vi "Determine Warning Bad One.vi"(6 "High":dbl, 7 "wind":dbl, 8 "error in (no error)":errorcluster, 9 "Low":dbl, 10 "Hi":dbl, 11 "Temp":dbl) -> (0 "error out":errorcluster, 1 "Stop":bool, 2 "text":string)   [LabVIEW 2010]
doc: "This is an example of inherited code that needs to be improved. Improve the VI for readability and maintainability, without changing the functionality."
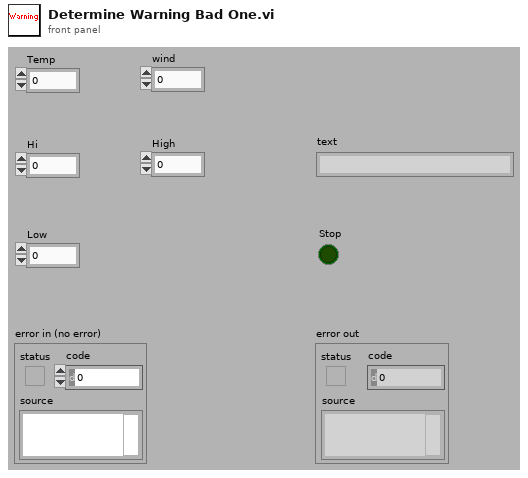
[diagram p1: front panel]
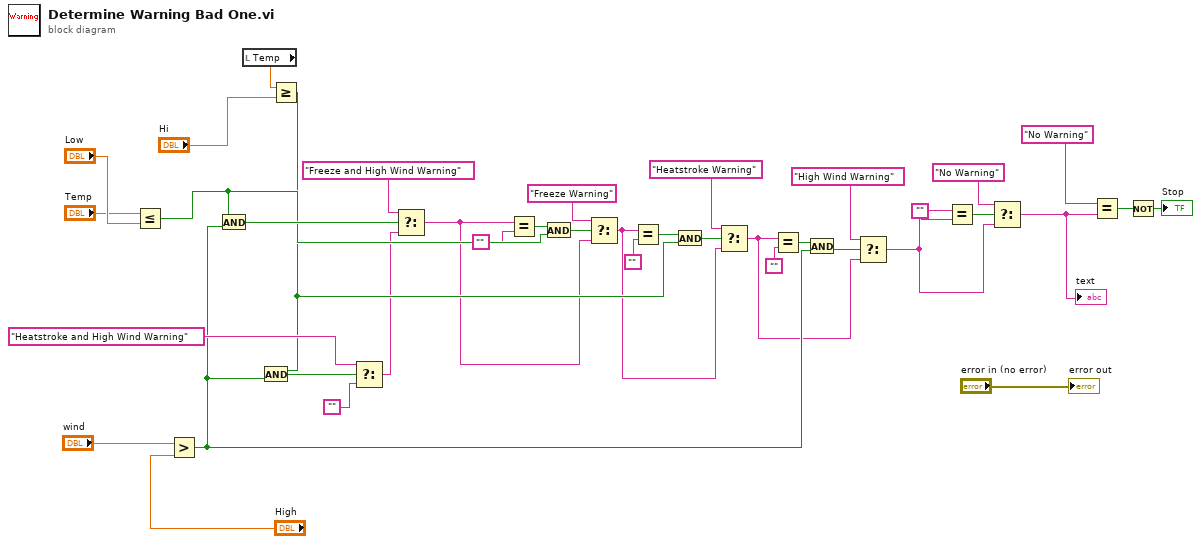
[diagram p0: block diagram]
diagram:
  n1 = Less Or Equal?(x="Temp", y="Low") -> (x <= y?=w27:bool)
  n2 = Greater?(x="wind", y="High") -> (0:w20:bool)
  n3 = And(x=w27, y=w20) -> (x .and. y?=w29:bool)
  n4 = local read "Temp"() -> (w7:dbl)
  n5 = Greater Or Equal?(x=w7, y="Hi") -> (x >= y?=w21:bool)
  n6 = And(x=w21, y=w20) -> (x .and. y?=w32:bool)
  n7 = Select(t="Heatstroke and High Wind Warning", s=w32, f="") -> (s? t:f=w14:string)
  n8 = Select(t="Freeze and High Wind Warning", s=w29, f=w14) -> (s? t:f=w13:string)
  n9 = Equal?(x=w13, y="") -> (x = y?=w28:bool)
  n10 = And(x=w28, y=w27) -> (x .and. y?=w26:bool)
  n11 = Select(t="Freeze Warning", s=w26, f=w13) -> (s? t:f=w11:string)
  n12 = Equal?(x=w11, y="") -> (x = y?=w23:bool)
  n13 = And(x=w23, y=w21) -> (x .and. y?=w24:bool)
  n14 = Select(t="Heatstroke Warning", s=w24, f=w11) -> (s? t:f=w12:string)
  n15 = Equal?(x=w12, y="") -> (x = y?=w19:bool)
  n16 = And(x=w19, y=w20) -> (x .and. y?=w18:bool)
  n17 = Select(t="High Wind Warning", s=w18, f=w12) -> (s? t:f=w9:string)
  n18 = Equal?(x=w9, y="") -> (x = y?=w15:bool)
  n19 = Select(t="No Warning" ("f"), s=w15, f=w9) -> (s? t:f=w38:string)
  "text" <- w38
  n20 = Equal?(x="No Warning" ("f"), y=w38) -> (x = y?=w2:bool)
  n21 = Not(x=w2) -> (.not. x?=→"Stop":bool)
  "error out" <- "error in (no error)"
